vi "client2.vi"() -> ()   [LabVIEW 2018]
panel:
  out "current time":timestamp
  out "time string":string
  out "date string":string
  in  "?":bool
  out "bytes written":i32=5
  in  "?":string
  out "Boolean":bool
  out "chat":string
  out "data out 2":string
  out "data out":string
  out "error out":errorcluster
  in  "?":bool
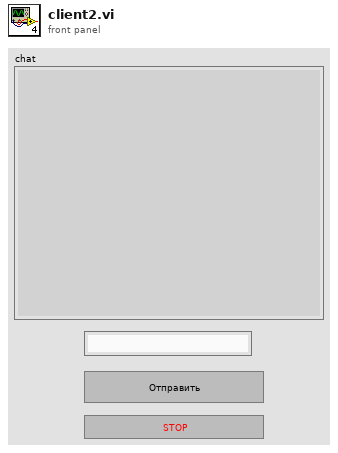
[diagram p1: front panel]
types:
  T1 = enum16{"Standard", "Buffered", "CRLF", "Immediate"}
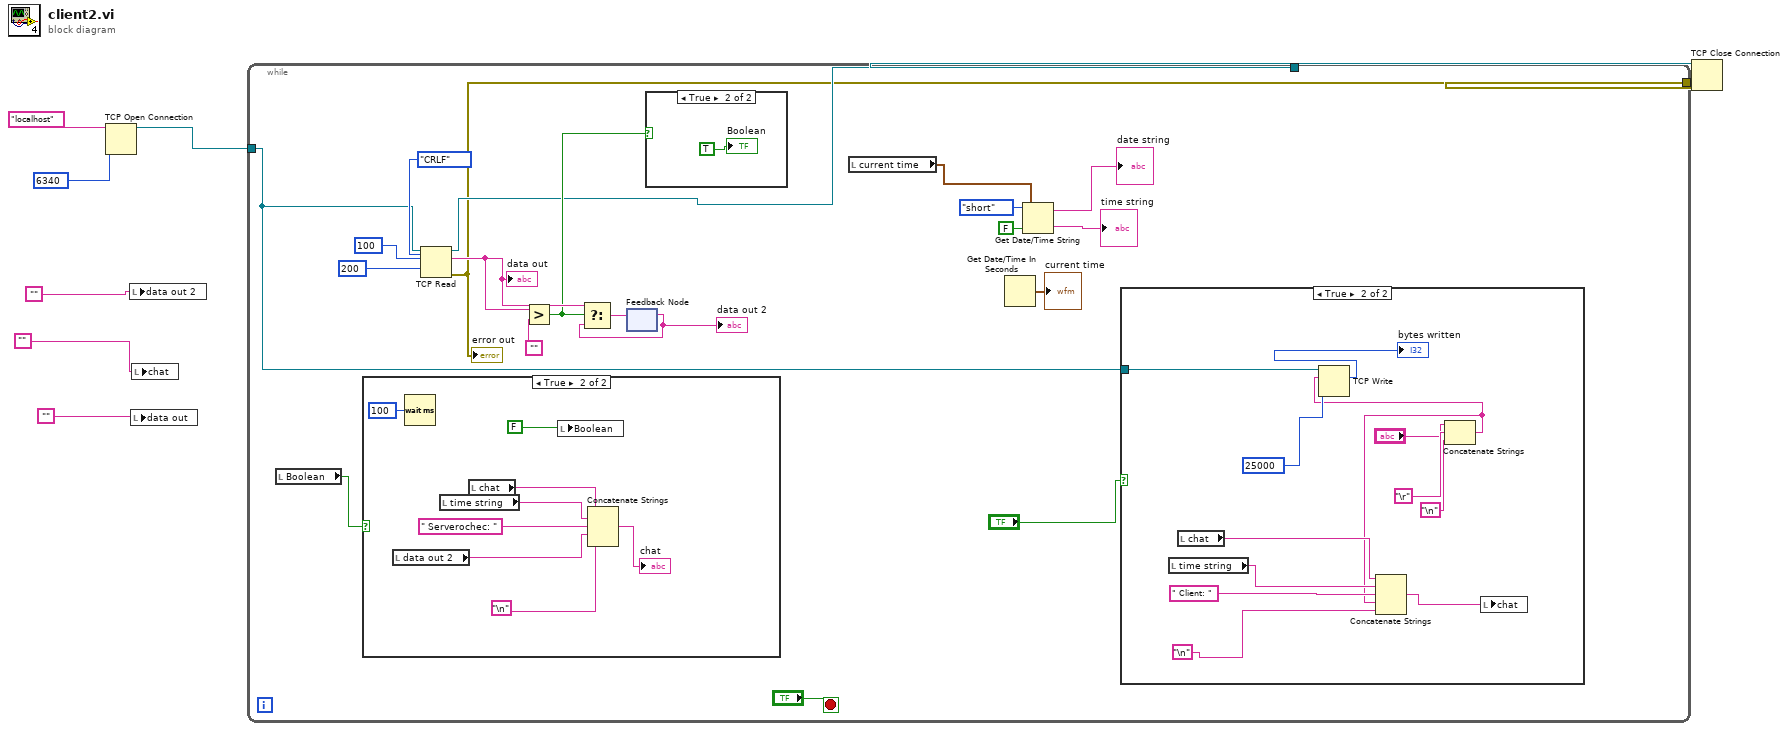
[diagram p0: block diagram]
diagram:
  n1 = TCP Open Connection(address="localhost", remote port or service name=u16 6340) -> (connection ID=w6:refnum<k5>)  [unwired: 3 in, 1 out]
  n2 = local write "data out 2"("") -> ()
  n3 = local write "data out"("") -> ()
  n4 = local write "chat"("") -> ()
  n5 = while {
    tunnel: w6 -> [w16]
    tunnel: [w17] -> w5
    tunnel: [w15] -> w2
    stop <- "?" stop-if-true
    n6 = local read "Boolean"() -> (w19:bool)
    n7 = case shown="True" w19 {
      frame False {
      }
      frame True {
        n8 = local read "data out 2"() -> (w42:string)
        n9 = Wait (ms)(milliseconds to wait=u32 100) -> ()  [unwired: 1 out]
        n10 = local read "time string"() -> (w44:string)
        n11 = local read "chat"() -> (w46:string)
        n12 = local write "Boolean"(FALSE ("Boolean")) -> ()
        n13 = Concatenate Strings(w46, w44, " Serverochec: " ("string"), w42, "\n") -> (→"chat":string)
      }
    }
    n14 = TCP Read(connection ID=w16, bytes to read=100, 7:T1."CRLF" ("mode (standard)"), 9:200 ("timeout ms (25000)")) -> (connection ID out=w17:refnum<k5>, data out=w24:string, error out=w15:errorcluster)  [unwired: 1 in]
    "error out" <- w15
    "data out" <- w24
    n15 = Greater?(x=w24, y="") -> (0:w20:bool)
    n16 = feedback #1() -> (w22:string)  [unwired: 1 in]
    "data out 2" <- w22
    n17 = Select(t=w24, s=w20, f=w22) -> (s? t:f=w23:string)
    n18 = feedback-in #1(w23) -> ()
    n19 = case shown="True" w20 {
      frame False {
      }
      frame True {
        "Boolean" <- TRUE ("Boolean")
      }
    }
    n20 = local read "current time"() -> (w9:timestamp)
    n21 = Get Date/Time In Seconds() -> (seconds since 1Jan1904=→"current time":timestamp)
    n22 = Get Date/Time String(date format (0)=enum16{"short", "long", "abbreviated"}."short", seconds (now)=w9, want seconds? (F)=FALSE) -> (date string=→"date string":string, time string=→"time string":string)
    n23 = case shown="True" "?" {
      tunnel: w16 -> [_ w36]
      frame False {
      }
      frame True {
        n24 = local read "time string"() -> (w33:string)
        n25 = local read "chat"() -> (w34:string)
        n26 = Concatenate Strings("?", "\r", "\n") -> (w29:string)
        n27 = TCP Write(connection ID=w36, data in=w29, 9:25000 ("timeout ms (25000)")) -> (bytes written=→"bytes written":i32)  [unwired: 1 in, 2 out]
        n28 = Concatenate Strings(w34, w33, " Client: " ("string"), w29, "\n") -> (w37:string)
        n29 = local write "chat"(w37) -> ()
      }
    }
  }
  n30 = TCP Close Connection(connection ID=w5, error in (no error)=w2) -> ()  [unwired: 1 in, 2 out]
